vi "FPGA_AIAverageBits.vi"(7 "Task":enum16{"Read", "Write"}(ring), 8 "error in (no error)":errorcluster, 10 "AverageBits in":u8[](array[numeric])=[0, 0, 0, 0, 0, 0, 0, 0], 11 "AI Reference in":T1) -> (0 "error out":errorcluster, 2 "AverageBits out":u8[](array[numeric]), 3 "AI Reference out":T1)   [LabVIEW 2017]
uses:
  <vilib>/Rock Robotics/SystemInterfaces/AI/FPGA_AIDevRef.ctl
  <vilib>/Utility/error.llb/Error Cluster From Error Code.vi
  <vilib>/rvi/errors/niLvFpgaAdjustHostInterfaceError.vi
  <vilib>/Rock Robotics/SystemInterfaces/System/FPGA_SystemFPGA Ref Global.vi
  <vilib>/rvi/interface/nirviReadWriteControl/nirviReadWriteControl.xnode
  <vilib>/Rock Robotics/SystemInterfaces/System/FPGA_SystemFRC FPGA Ref.ctl
  <vilib>/rvi/interface/Simulation/niFpgaSimulationCallBeginRW.vi
  NiFpgaLv.dll
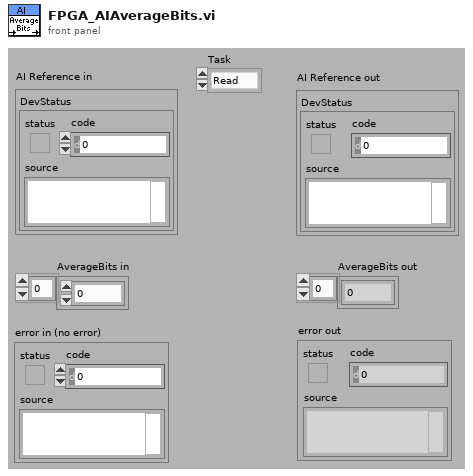
[diagram p1: front panel]
types:
  T1 = typedef "FPGA_AIDevRef.ctl" = cluster{"DevStatus":errorcluster}
  T2 = typedef "FPGA_SystemFRC FPGA Ref.ctl" = refnum<k20>
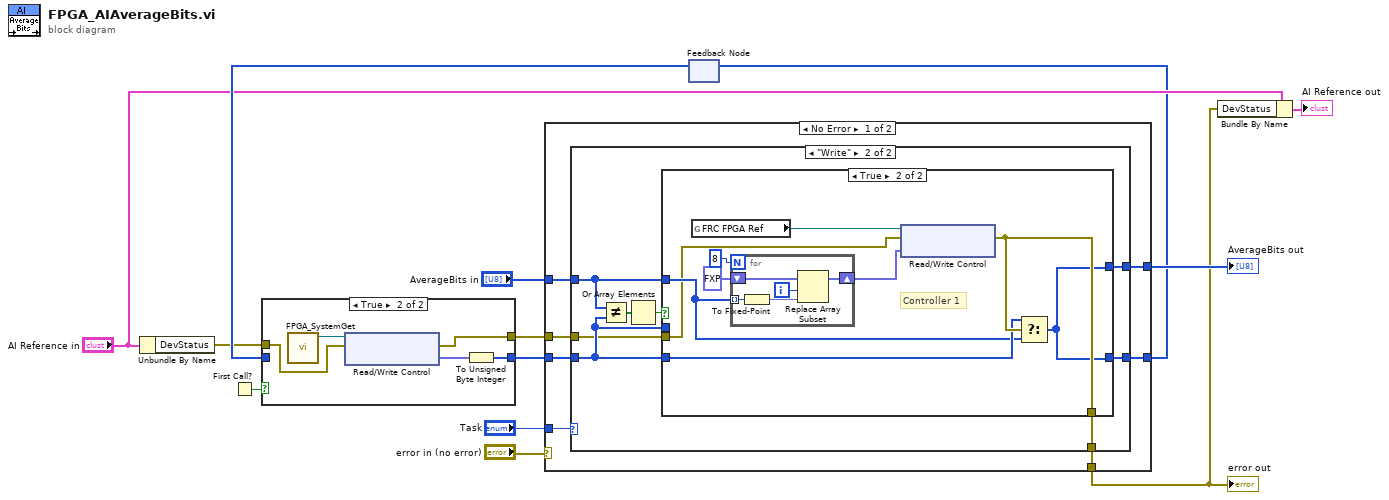
[diagram p0: block diagram]
diagram:
  n1 = Unbundle By Name("AI Reference in") -> ("DevStatus"=w3:errorcluster)
  n2 = First Call?() -> (First Call?: T/F=w13:bool)
  n3 = feedback #1() -> (w12:u8[])  [unwired: 1 out]
  n4 = case shown="True" w13 {
    tunnel: [w14 w17] -> w2
    tunnel: [w15 w19] -> w10
    tunnel: w12 -> [w15 _]
    tunnel: w3 -> [w14 w16]
    frame False {
    }
    frame True {
      n5 = call <vilib>:"FPGA_SystemGet.vi"() -> ("FRC FPGA Ref"=w18:T2)  [unwired: 2 in, 9 out]
      n6 = xnode "Read/Write Control"("FPGA VI Reference In"=w18, "error in"=w16) -> ("error out"=w17:errorcluster, "AI.AverageBits"=w20:fxp<+,4,4>[])  [unwired: 1 out]
      n7 = To Unsigned Byte Integer(number=w20) -> (unsigned 8bit integer=w19:u8[])
    }
  }
  n8 = case shown="No Error" "error in (no error)" {
    selector: "error in (no error)" -> [_ w55]
    tunnel: "Task" -> [w27 _]
    tunnel: w10 -> [w26 w56]
    tunnel: "AverageBits in" -> [w25 _]
    tunnel: [w24 w55] -> w1
    tunnel: [w23 w56] -> w4
    tunnel: [w22 _] -> w7
    tunnel: w2 -> [w21 _]
    frame No Error {
      n9 = case shown="\"Write\"" w27 {
        tunnel: w26 -> [w29 w31]
        tunnel: w25 -> [_ w34]
        tunnel: [w28 w37] -> w24
        tunnel: [w29 w36] -> w23
        tunnel: [w29 w35] -> w22
        tunnel: w21 -> [w28 w30]
        frame "Read" {
        }
        frame "Write" {
          n10 = Not Equal?(x=w34, y=w31) -> (x != y?=w33:bool[])
          n11 = Or Array Elements(Boolean array=w33) -> (logical OR=w32:bool)
          n12 = case shown="True" w32 {
            tunnel: [w40 w46] -> w37
            tunnel: [w39 w45] -> w36
            tunnel: [w38 w45] -> w35
            tunnel: w31 -> [w39 w44]
            tunnel: w34 -> [_ w43]
            tunnel: w30 -> [w40 w41]
            tunnel: w31 -> [w38 _]
            frame False {
              # "AverageBits In matches current array\nso no need to write anything"
            }
            frame True {
              # "Controller 1"
              n13 = global read "FPGA_SystemFPGA Ref Global.vi" "FRC FPGA Ref"() -> (w42:T2)
              n14 = for {
                N: 8 -> [_]
                tunnel: w43 -> [w54] mode=indexing
                shift-right: [w52] -> w47
                shift-left: fxp<+,4,4>[] [0.0, 0.0, 0.0, 0.0, 0.0, 0.0, 0.0, 0.0] ("AI0.AverageBits") -> [w53]
                i -> [w50]
                n15 = To Fixed-Point(number=w54) -> (fixed-point=w51:fxp<+,4,4>)  [unwired: 1 out]
                n16 = Replace Array Subset(array=w53, new element=w51, index=w50) -> (w52:fxp<+,4,4>[])
              }
              n17 = xnode "Read/Write Control"("FPGA VI Reference In"=w42, "error in"=w41, "AI.AverageBits"=w47) -> ("error out"=w46:errorcluster)  [unwired: 1 out]
              n18 = Select(t=w44, s=w46, f=w43) -> (s? t:f=w45:u8[])
            }
          }
        }
      }
    }
    frame Error {
    }
  }
  "AverageBits out" <- w7
  "error out" <- w1
  n19 = feedback-in #1(w4) -> ()
  n20 = Bundle By Name(cluster="AI Reference in", "DevStatus"=w1) -> (→"AI Reference out":T1)
